vi "FindDecoration.vi"(5 "Decoration in":refnum<class "Decoration.lvclass">, 6 "error in":errorcluster, 9 "Page in":refnum<class "Page.lvclass">) -> (0 "error out":errorcluster, 3 "Page out":refnum<class "Page.lvclass">, 4 "On page":bool)   [LabVIEW 2014, in "Raspberry Pi Compatible Compiler for LabVIEW.lvlib" / "Page.lvclass"]
uses:
  Page.lvclass
  Decoration/Decoration.lvclass
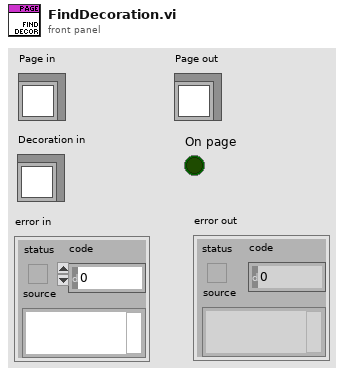
[diagram p1: front panel]
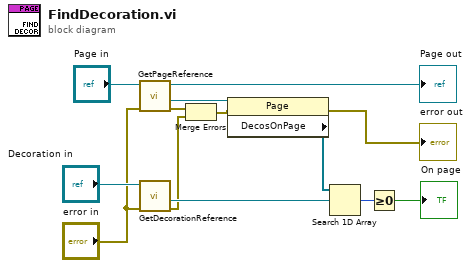
[diagram p0: block diagram]
diagram:
  n1 = call "GetPageReference.vi"("error in"="error in", "Page in"="Page in") -> ("error out"=w2:errorcluster, "page reference"=w10:refnum<vi>, "Page out"=→"Page out":refnum<class "Page.lvclass">)  [unwired: 7 in]
  n2 = call "GetDecorationReference.vi"("error in"="error in", "Decoration in"="Decoration in") -> ("error out"=w3:errorcluster, "Decoration reference"=w8:refnum<vi>)  [unwired: 7 in, 1 out]
  n3 = Merge Errors(w2, w3) -> (w1:errorcluster)
  n4 = property class="Page"(reference=w10, error in=w1) -> (error out=→"error out":errorcluster, "DecosOnPage"=w9:refnum<vi>[])  [unwired: 1 out]
  n5 = Search 1D Array(1D array=w9, element=w8) -> (index of element=w6:i32)  [unwired: 1 in]
  n6 = Greater Or Equal To 0?(x=w6) -> (x >= 0?=→"On page":bool)
